vi "34_Roberts_cross.vi"() -> ()   [LabVIEW 2018]
uses:
  <vilib>/Analysis/2dsp.llb/2D Convolution (DBL).vi
  <vilib>/vision/NI_Vision_Development_Module.lvlib
  <vilib>/Analysis/NI_AALPro.lvlib
panel:
  in  "<adj":u8(slide) scale=0.0..255.0
  in  ">adj":u8(slide)=255 scale=0.0..255.0
  in  "adj":u8(slide)=22 scale=0.0..50.0
  out "new":T1(plugin-control)
  out "Array":u8[][](array[numeric])
  out "Image 2":T1(plugin-control)
  out "Image Pixels (U8)":u8[][](array[numeric])
  in  "stop":bool
  out "Image":T1(plugin-control)
  # "邊緣檢測 Roberts_cross"
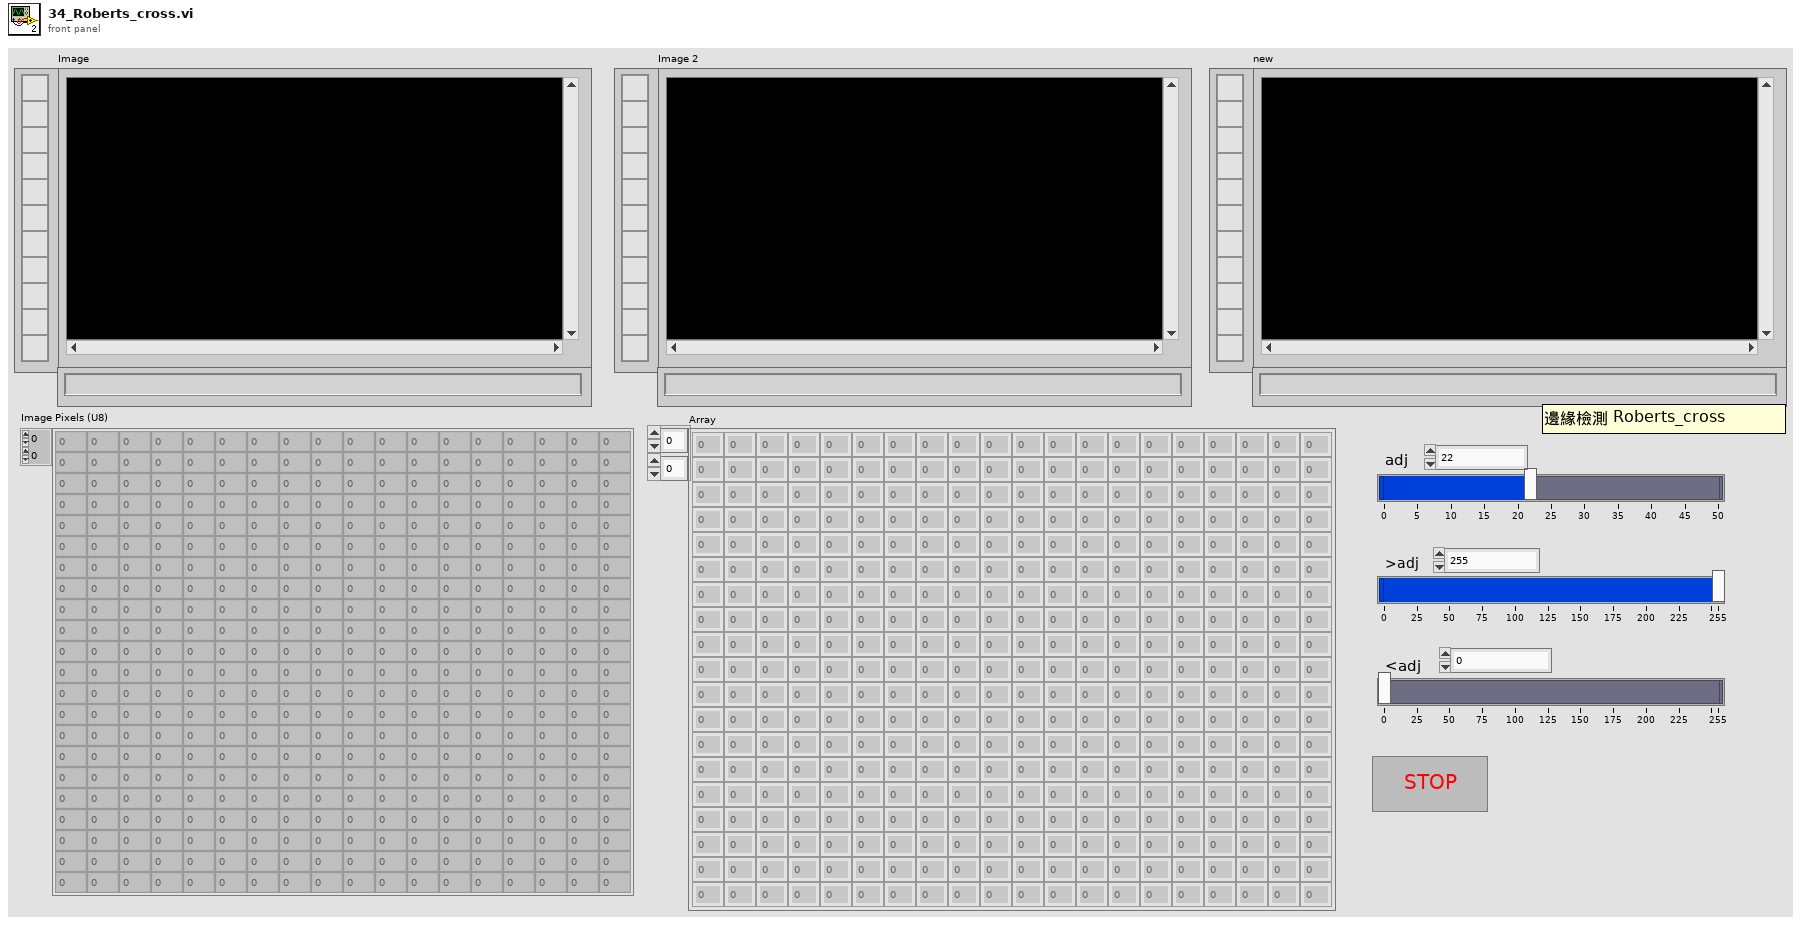
[diagram p1: front panel]
types:
  T1 = typedef "IMAQ Image.ctl" = refnum<image>
  T2 = typedef "Image Type" = u32
  T3 = cluster{"Global Rectangle":i32[], "Contours":cluster{"Contour Type":u32, "ROI Type":u32, "Points":i32[]}[]}
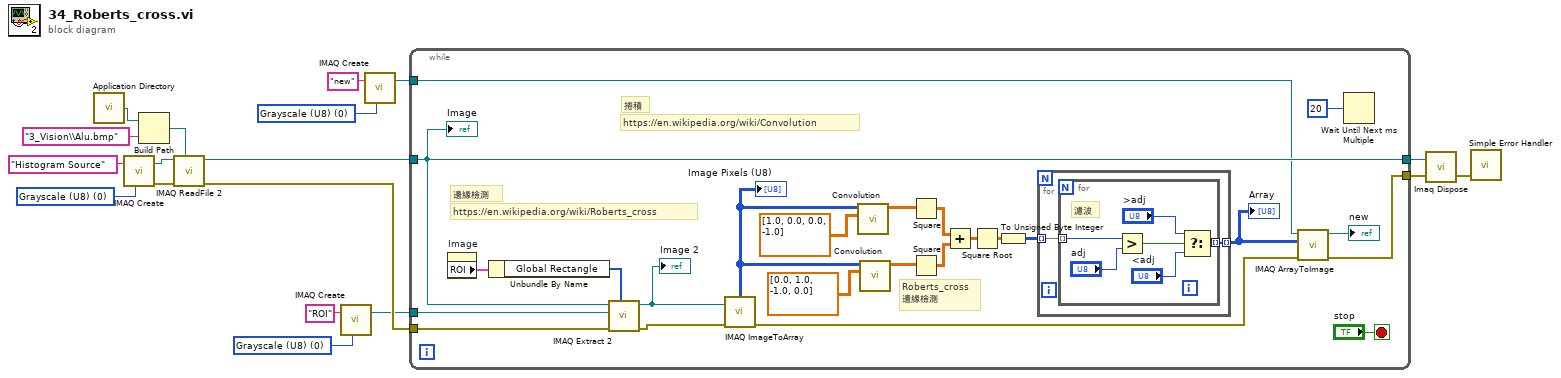
[diagram p0: block diagram]
diagram:
  w2 = T2 0 items=["Grayscale (U8)", "Grayscale (I16)", "Grayscale (SGL)", "Complex (CSG)", "RGB (U32)", "HSL (U32)", "RGB (U64)", "Grayscale (U16)"] ("Image Type")
  w7 = T2 0 items=["Grayscale (U8)", "Grayscale (I16)", "Grayscale (SGL)", "Complex (CSG)", "RGB (U32)", "HSL (U32)", "RGB (U64)", "Grayscale (U16)"] ("Image Type")
  w8 = T2 0 items=["Grayscale (U8)", "Grayscale (I16)", "Grayscale (SGL)", "Complex (CSG)", "RGB (U32)", "HSL (U32)", "RGB (U64)", "Grayscale (U16)"] ("Image Type")
  n1 = call <vilib>:"Application Directory.vi"() -> ("Application Directory"=w10:path)
  n2 = call "IMAQ Create"("Image Name"="Histogram Source", "Image Type"=w8) -> ("New Image"=w18:T1, "error out"=w17:errorcluster)  [unwired: 3 in]
  n3 = Build Path(base path=w10, name or relative path="3_Vision\\Alu.bmp") -> (appended path=w11:path)
  n4 = call "IMAQ ReadFile 2"("File Path"=w11, "error in (no error)"=w17, "Image"=w18) -> ("error out"=w13:errorcluster, "Image Out"=w15:T1)  [unwired: 4 in, 3 out]
  n5 = call "IMAQ Create"("Image Name"="ROI", "Image Type"=w7) -> ("New Image"=w5:T1)  [unwired: 3 in, 1 out]
  n6 = call "IMAQ Create"("Image Name"="new", "Image Type"=w2) -> ("New Image"=w1:T1)  [unwired: 3 in, 1 out]
  n7 = while {
    tunnel: w15 -> [w39]
    tunnel: [w39] -> w14
    tunnel: w13 -> [w36]
    tunnel: w5 -> [w38]
    tunnel: [w30] -> w4
    tunnel: w1 -> [w33]
    stop <- "stop" stop-if-true
    # "邊緣檢測"
    # "https://en.wikipedia.org/wiki/Roberts_cross"
    # "捲積"
    # "https://en.wikipedia.org/wiki/Convolution"
    # "Roberts_cross\n邊緣檢測"
    n8 = property on="Image" class="ImageControl"() -> ("ROI"=w40:T3)  [unwired: 2 in, 2 out]
    n9 = Unbundle By Name "Unbundle By Name"(w40) -> ("Global Rectangle"=w37:i32[])
    n10 = call "IMAQ Extract 2"("Optional Rectangle"=w37, "error in (no error)"=w36, "Image Dst"=w38, "Image Src"=w39) -> ("error out"=w34:errorcluster, "Image Dst Out"=w35:T1)  [unwired: 6 in]
    "Image 2" <- w35
    n11 = call "IMAQ ImageToArray"("error in (no error)"=w34, "Image"=w35) -> ("error out"=w31:errorcluster, "Image Pixels (U8)"=w25:u8[][])  [unwired: 2 in, 3 out]
    "Image Pixels (U8)" <- w25
    n12 = call-poly <vilib>:"Convolution.vi"("Y"=dbl[][] [[1.0, 0.0], [0.0, -1.0]], "X"=w25) -> ("X * Y"=w28:dbl[][])  [unwired: 8 in, 1 out]
    n13 = call-poly <vilib>:"Convolution.vi"("Y"=dbl[][] [[0.0, 1.0], [-1.0, 0.0]], "X"=w25) -> ("X * Y"=w26:dbl[][])  [unwired: 8 in, 1 out]
    n14 = Square(x=w28) -> (x^2=w23:dbl[][])
    n15 = Square(x=w26) -> (x^2=w22:dbl[][])
    n16 = Add(x=w23, y=w22) -> (x+y=w24:dbl[][])
    n17 = Square Root(x=w24) -> (sqrt(x)=w21:dbl[][])
    n18 = To Unsigned Byte Integer(number=w21) -> (unsigned 8bit integer=w20:u8[][])
    n19 = for {
      tunnel: w20 -> [w44] mode=indexing
      tunnel: [w43] -> w19 mode=indexing
      n20 = for {
        tunnel: w44 -> [w50] mode=indexing
        tunnel: [w45] -> w43 mode=indexing
        # "濾波"
        n21 = Greater?(x=w50, y="adj") -> (0:w48:bool)
        n22 = Select(t=">adj", s=w48, f="<adj") -> (s? t:f=w45:u8)
      }
    }
    "Array" <- w19
    n23 = call "IMAQ ArrayToImage"("error in (no error)"=w31, "Image Pixels (U8)"=w19, "Image"=w33) -> ("error out"=w30:errorcluster, "Image Out"=→"new":T1)  [unwired: 7 in]
    n24 = Wait Until Next ms Multiple(millisecond multiple=u32 20) -> ()  [unwired: 1 out]
    "Image" <- w39
  }
  n25 = call "Imaq Dispose"("Image"=w14, "error in (no error)"=w4) -> ("error out"=w12:errorcluster)  [unwired: 4 in]
  n26 = call <vilib>:"Simple Error Handler.vi"("error in (no error)"=w12) -> ()  [unwired: 4 in, 5 out]
